vi "gameFunc.vi"(8 "Error In":errorcluster) -> (0 "Error Out":errorcluster)   [LabVIEW 2014]
uses:
  C_Library/scanf string.vi
  C_Library/C Basic Lib.lvlib
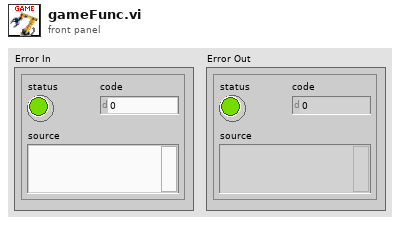
[diagram p1: front panel]
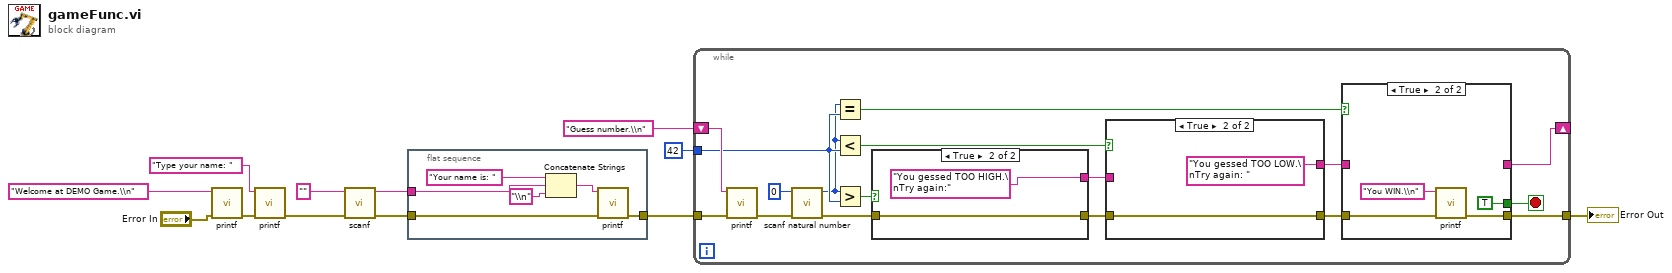
[diagram p0: block diagram]
diagram:
  n1 = call "printf.vi"("Error In"="Error In", "String"="Welcome at DEMO Game.\\n") -> ("Error Out"=w10:errorcluster)  [unwired: 9 in]
  n2 = call "printf.vi"("Error In"=w10, "String"="Type your name: ") -> ("Error Out"=w8:errorcluster)  [unwired: 9 in]
  n3 = call-poly "scanf.vi"("Error In"=w8, "String in"="" ("String")) -> ("Error Out"=w7:errorcluster, "String out"=w1:string)  [unwired: 8 in]
  n4 = flat-sequence {
    tunnel: w7 -> [w18]
    tunnel: w1 -> [w17]
    tunnel: [w14] -> w5
    frame #0 {
      n5 = Concatenate Strings("Your name is: " ("string"), w17, "\\n" ("string")) -> (w15:string)
      n6 = call "printf.vi"("Error In"=w18, "String"=w15) -> ("Error Out"=w14:errorcluster)  [unwired: 9 in]
    }
  }
  n7 = while {
    tunnel: w5 -> [w35]
    tunnel: 42 -> [w21]
    tunnel: [w25] -> w3
    shift-right: [w24] -> _
    shift-left: "Guess number.\\n" ("String") -> [w23]
    stop <- w29 stop-if-true
    n8 = call "printf.vi"("Error In"=w35, "String"=w23) -> ("Error Out"=w34:errorcluster)  [unwired: 9 in]
    n9 = call "scanf natural number.vi"("Error In"=w34, "natural number (decadic)"=0) -> ("Error Out"=w33:errorcluster, "number out"=w19:i32)  [unwired: 8 in]
    n10 = Equal?(x=w19, y=w21) -> (x = y?=w27:bool)
    n11 = Less?(x=w19, y=w21) -> (x < y?=w31:bool)
    n12 = Greater?(x=w19, y=w21) -> (0:w22:bool)
    n13 = case shown="True" w22 {
      tunnel: w33 -> [w46 w48]
      tunnel: [w46 w48] -> w32
      tunnel: [_ "You gessed TOO HIGH.\nTry again:" ("String")] -> w28
      frame False {
      }
      frame True {
      }
    }
    n14 = case shown="True" w31 {
      tunnel: w32 -> [w42 w45]
      tunnel: [w42 w45] -> w30
      tunnel: [w43 "You gessed TOO LOW.\nTry again: " ("String")] -> w26
      tunnel: w28 -> [w43 _]
      frame False {
      }
      frame True {
      }
    }
    n15 = case shown="True" w27 {
      tunnel: w30 -> [w36 w38]
      tunnel: [w36 w40] -> w25
      tunnel: [w37 _] -> w24
      tunnel: [_ TRUE] -> w29
      tunnel: w26 -> [w37 _]
      frame False {
      }
      frame True {
        n16 = call "printf.vi"("Error In"=w38, "String"="You WIN.\\n") -> ("Error Out"=w40:errorcluster)  [unwired: 9 in]
      }
    }
  }
  "Error Out" <- w3
